vi "Overall_Test_V2.vi"() -> ()   [LabVIEW 2020]
uses:
  <vilib>/DAQmx/read.llb/DAQmx Read (Digital Bool 1Line 1Point).vi
  <vilib>/DAQmx/read.llb/DAQmx Read (Analog 1D Wfm NChan NSamp).vi
  <vilib>/Utility/file.llb/Read Delimited Spreadsheet (DBL).vi
  <vilib>/DAQmx/create/channels.llb/DAQmx Create Channel (AI-Acceleration-Accelerometer).vi
  <vilib>/DAQmx/configure/timing.llb/DAQmx Timing (Sample Clock).vi
  <vilib>/DAQmx/create/channels.llb/DAQmx Create Channel (DI-Digital Input).vi
  <vilib>/DAQmx/miscellaneous.llb/DAQmx Fill In Error Info.vi
  <vilib>/express/express analysis/Spectral/Block/exnSpectralBlock spectral measurements RMS poly.vi
  <vilib>/express/express analysis/Spectral/Block/exnSpectralBlock spectral measurements RMS array WFM.vi
  <vilib>/express/express analysis/Spectral/XNode/ExpressSpectralMeasurementsBlockNode.xnode
  <resource>/objmgr/daqmx.rc
panel:
  out "data":waveform(dbl)[](graph)
  in  "stop":bool
  out "Trigger":bool
  out "data 2":cluster{"f0":dbl, "df":dbl, "magnitude":dbl[]}[](graph) caption="data"
  in  "Scale":dbl
  out "first row":dbl[](array[numeric])
  out "Input":waveform(dbl)(graph)
  in  "file to run":path=path "C:/Users/Puja/Desktop/Labview(PC)/Input_Signal/Sine_wave_data_without_time/data1_w1_NT_1per.txt"
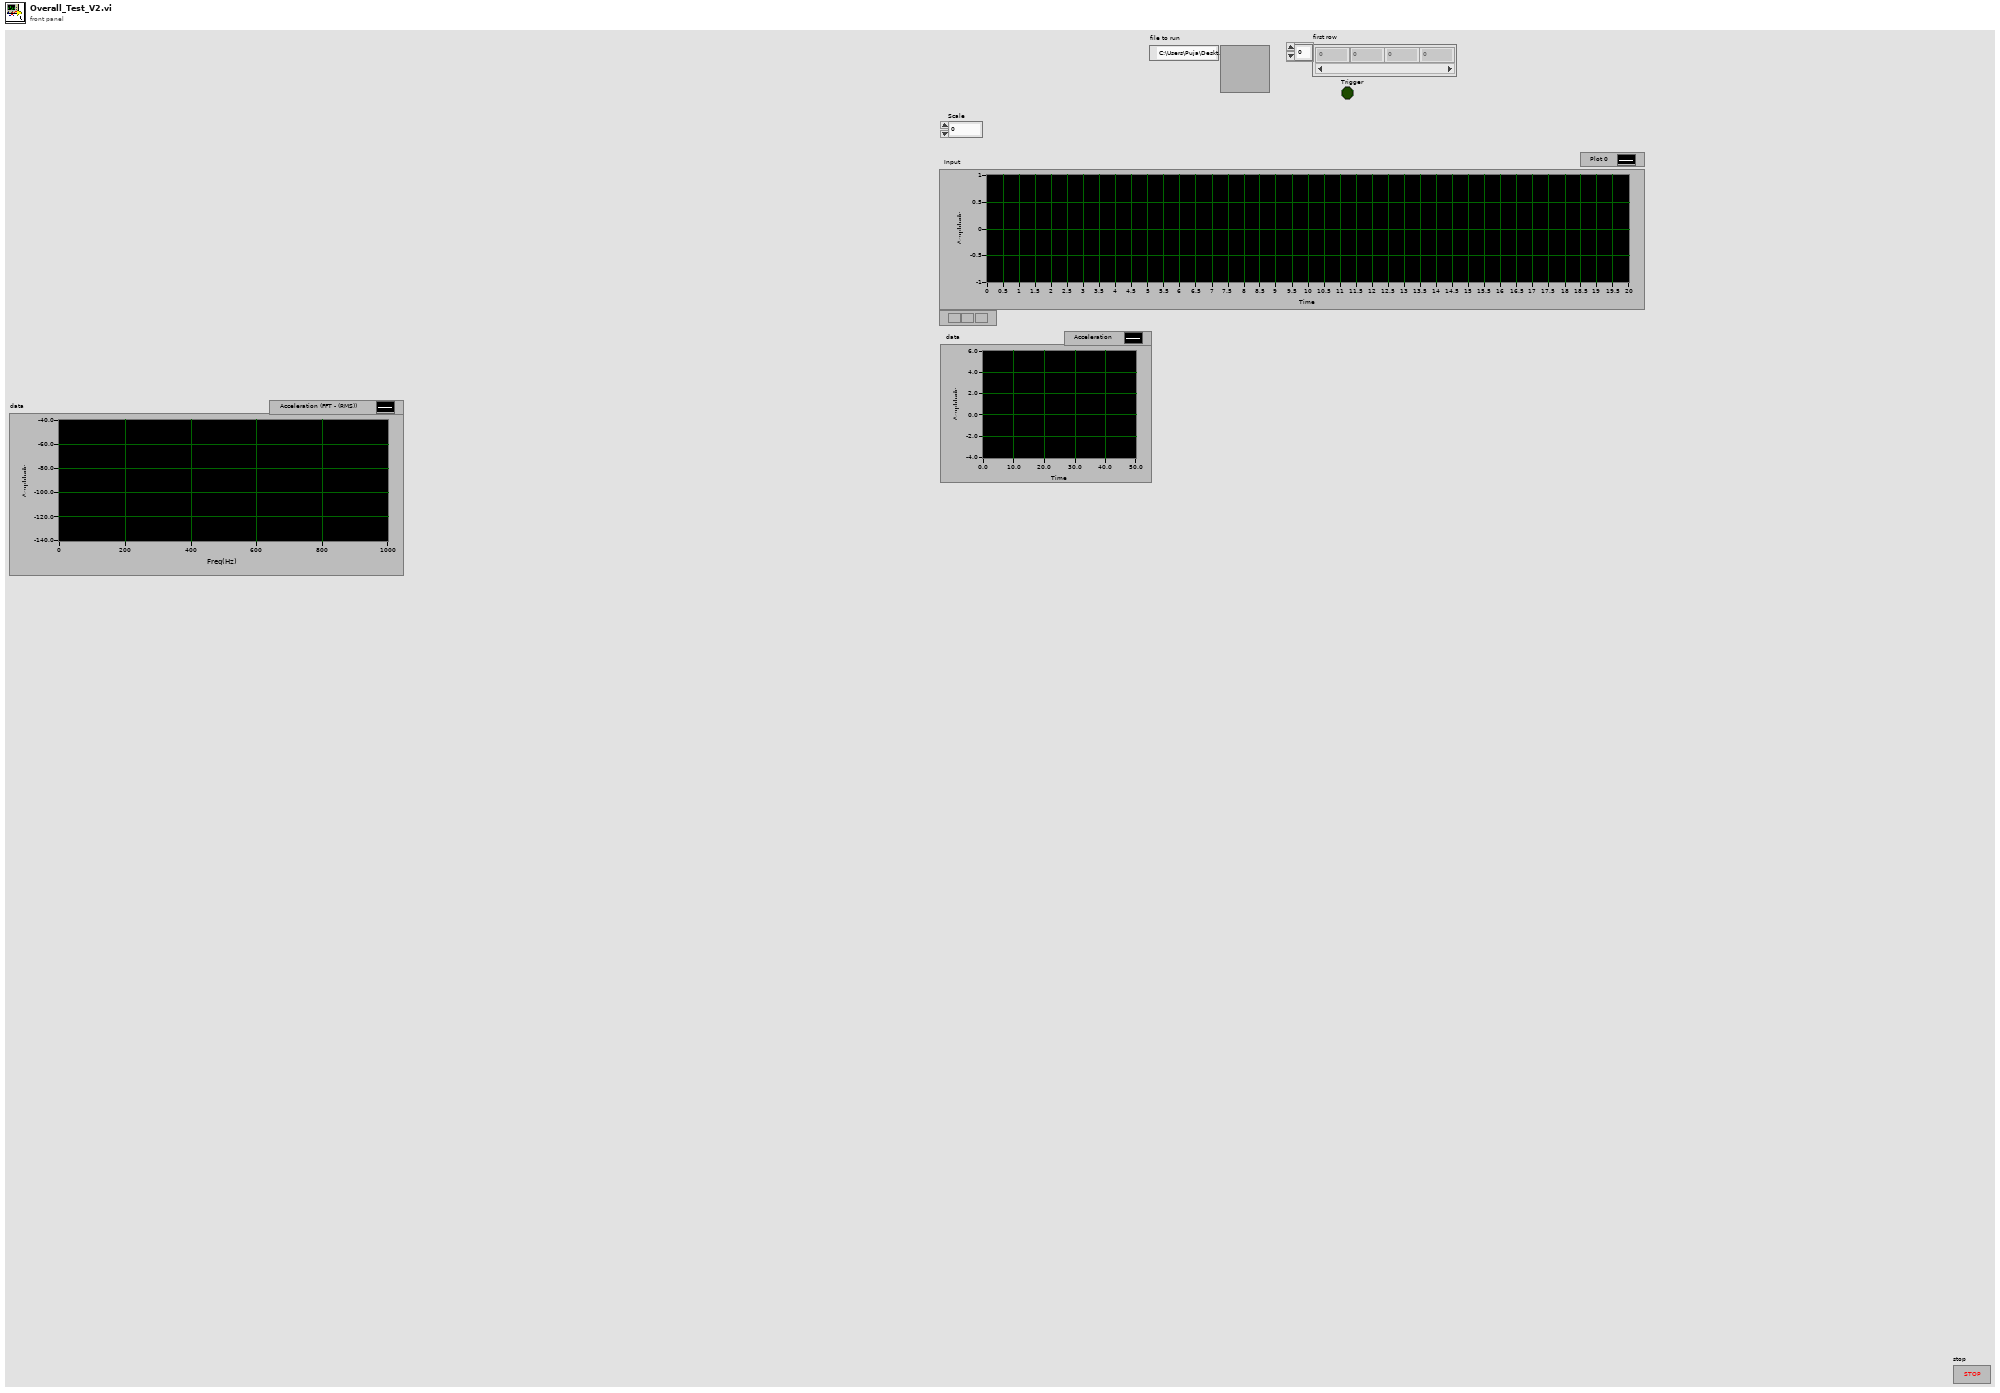
[diagram p1: front panel]
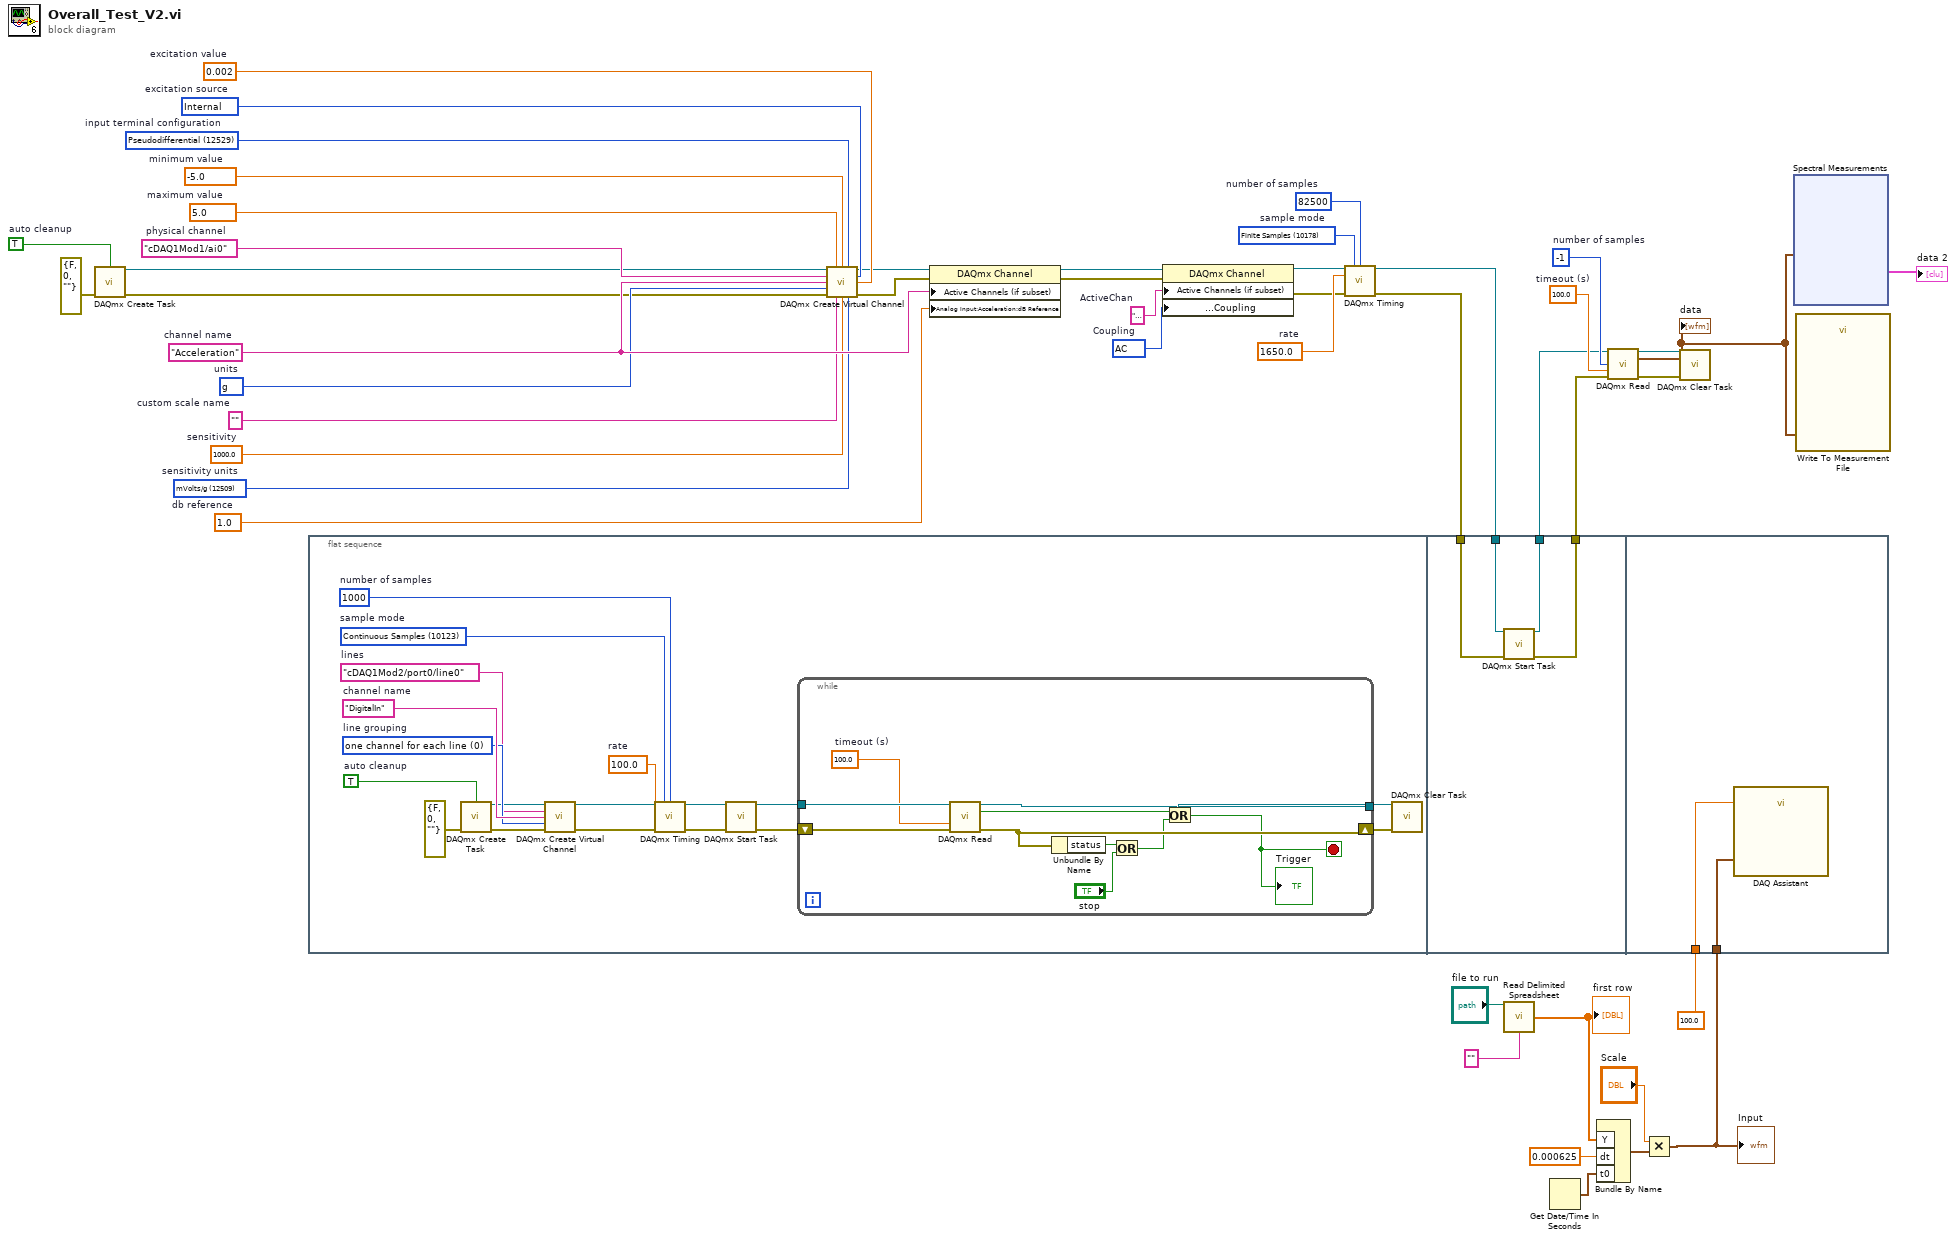
[diagram p0: block diagram]
diagram:
  w33 = 10178 items=["Finite Samples"=10178, "Continuous Samples"=10123, "Hardware Timed Single Point"=12522]  # sample mode
  w32 = 82500  # number of samples
  w31 = 1650.0  # rate
  w27 = 10045 items=["AC"=10045, "DC"=10050, "GND"=10066]  # Coupling
  w26 = "Acceleration"  # ActiveChan
  w24 = 1.0  # db reference
  w21 = 10186 items=["g"=10186, "m/s^2"=12470, "From Custom Scale"=10065]  # units
  w20 = 12529 items=["default"=-1, "RSE"=10083, "NRSE"=10078, "Differential"=10106, "Pseudodifferential"=12529]  # input terminal configuration
  w19 = 10200 items=["Internal"=10200, "External"=10167, "None"=10230]  # excitation source
  w18 = 0.002  # excitation value
  w17 = 12509 items=["mVolts/g"=12509, "Volts/g"=12510]  # sensitivity units
  w16 = 1000.0  # sensitivity
  w25 = "Acceleration"  # channel name
  w14 = ""  # custom scale name
  w13 = -5.0  # minimum value
  w12 = 5.0  # maximum value
  w11 = "cDAQ1Mod1/ai0"  # physical channel
  w9 = TRUE  # auto cleanup
  w37 = 100.0  # timeout (s)
  w38 = -1  # number of samples
  n1 = call <vilib>:"DAQmx Create Task.vi"("auto cleanup"=w9, "error in"=errorcluster {"status"=FALSE, "code"=0, "source"=""}) -> ("task out"=w10:refnum<k21>, "error out"=w8:errorcluster)  [unwired: 12 in]
  n2 = flat-sequence {
    tunnel: w7 -> [w78]
    tunnel: w6 -> [w77]
    tunnel: [w76] -> w5
    tunnel: [w75] -> w4
    tunnel: w2 -> [w80]
    tunnel: 100.0 ("timeout (s)") -> [w79]
    frame #0 {
      w57 = 10123 items=["Finite Samples"=10178, "Continuous Samples"=10123, "Hardware Timed Single Point"=12522]  # sample mode
      w56 = 1000  # number of samples
      w55 = 100.0  # rate
      w51 = 0 items=["one channel for each line", "one channel for all lines"]  # line grouping
      w52 = "DigitalIn"  # channel name
      w50 = "cDAQ1Mod2/port0/line0"  # lines
      w48 = TRUE  # auto cleanup
      n3 = call <vilib>:"DAQmx Create Task.vi"("auto cleanup"=w48, "error in"=errorcluster {"status"=FALSE, "code"=0, "source"=""}) -> ("task out"=w49:refnum<k21>, "error out"=w47:errorcluster)  [unwired: 12 in]
      n4 = call-poly <vilib>:"DAQmx Create Virtual Channel.vi"("task in"=w49, "lines"=w50, "name to assign"=w52, "line grouping"=w51, "error in"=w47) -> ("task out"=w54:refnum<k21>, "error out"=w53:errorcluster)  [unwired: 9 in]
      n5 = call-poly <vilib>:"DAQmx Timing.vi"("task/channels in"=w54, "sample mode"=w57, "samples per channel"=w56, "rate"=w55, "error in"=w53) -> ("task out"=w60:refnum<k21>, "error out"=w59:errorcluster)  [unwired: 9 in]
      n6 = call <vilib>:"DAQmx Start Task.vi"("task/channels in"=w60, "error in"=w59) -> ("task out"=w64:refnum<k21>, "error out"=w63:errorcluster)  [unwired: 12 in]
      n7 = while {
        tunnel: w64 -> [w74]
        tunnel: [w72] -> w61
        shift-right: [w70] -> w62
        shift-left: w63 -> [w73]
        stop <- w66 stop-if-true
        w68 = 100.0  # timeout (s)
        n8 = call-poly <vilib>:"DAQmx Read.vi"("task/channels in"=w74, "timeout"=w68, "error in"=w73) -> ("task out"=w72:refnum<k21>, "data"=w65:bool, "error out"=w70:errorcluster)  [unwired: 10 in]
        n9 = Unbundle By Name(w70) -> ("status"=w71:bool)
        n10 = Or(x=w71, y="stop") -> (x .or. y?=w67:bool)
        n11 = Or(x=w65, y=w67) -> (x .or. y?=w66:bool)
        "Trigger" <- w66
      }
      n12 = call <vilib>:"DAQmx Clear Task.vi"("task in"=w61, "error in"=w62) -> ()  [unwired: 13 in, 1 out]
    }
    frame #1 {
      n13 = call <vilib>:"DAQmx Start Task.vi"("task/channels in"=w78, "error in"=w77) -> ("task out"=w76:refnum<k21>, "error out"=w75:errorcluster)  [unwired: 12 in]
    }
    frame #2 {
      n14 = call "DAQ Assistant"("data"=w80, "timeout (s)"=w79) -> ()  [unwired: 16 in, 2 out]
    }
  }
  n15 = call-poly <vilib>:"DAQmx Create Virtual Channel.vi"("task in"=w10, "maximum value"=w12, "minimum value"=w13, "input terminal configuration"=w20, "physical channels"=w11, "current excitation source"=w19, "name to assign"=w25, "current excitation value"=w18, "units"=w21, "error in"=w8, "custom scale name"=w14, "sensitivity"=w16, "sensitivity units"=w17) -> ("task out"=w15:refnum<k21>, "error out"=w22:errorcluster)  [unwired: 1 in]
  n16 = property class="DAQmx Channel"(reference=w15, error in=w22, "Active Channels (if subset)"=w25, "Analog Input:Acceleration:dB Reference"=w24) -> (reference out=w29:refnum<k21>, error out=w23:errorcluster)
  n17 = property class="DAQmx Channel"(reference=w29, error in=w23, "Active Channels (if subset)"=w26, "Analog Input:General Properties:Input Configuration:Coupling"=w27) -> (reference out=w30:refnum<k21>, error out=w28:errorcluster)
  n18 = call-poly <vilib>:"DAQmx Timing.vi"("task/channels in"=w30, "sample mode"=w33, "samples per channel"=w32, "rate"=w31, "error in"=w28) -> ("task out"=w7:refnum<k21>, "error out"=w6:errorcluster)  [unwired: 9 in]
  n19 = call-poly <vilib>:"Read Delimited Spreadsheet.vi"("file path (dialog if empty)"="file to run", "delimiter (\\t)"="") -> ("first row"=w45:dbl[])  [unwired: 8 in, 5 out]
  "first row" <- w45
  n20 = Get Date/Time In Seconds() -> (seconds since 1Jan1904=w43:timestamp)
  n21 = Bundle By Name("Y"=w45, "dt"=0.000625, "t0"=w43) -> (w41:waveform(dbl))  [unwired: 1 in]
  n22 = call-poly <vilib>:"DAQmx Read.vi"("task/channels in"=w5, "number of samples per channel"=w38, "timeout"=w37, "error in"=w4) -> ("task out"=w35:refnum<k21>, "data"=w3:waveform(dbl)[], "error out"=w36:errorcluster)  [unwired: 9 in]
  "data" <- w3
  n23 = Multiply(x="Scale", y=w41) -> (x*y=w2:waveform(dbl))
  "Input" <- w2
  n24 = call <vilib>:"DAQmx Clear Task.vi"("task in"=w35, "error in"=w36) -> ()  [unwired: 13 in, 1 out]
  n25 = xnode "Spectral Measurements"("Signals"=w3) -> ("FFT - (RMS)"=→"data 2":cluster{"f0":dbl, "df":dbl, "magnitude":dbl[]}[])  [unwired: 1 in, 2 out]
  n26 = call "Write To Measurement File"("Signals"=w3) -> ()  [unwired: 16 in, 3 out]
